vi "autonSample.vi"(0 "Auton Array":dbl[][](array[numeric]), 5 "LeftEncoder":dbl, 7 "RightEncoder":dbl, 11 "MeasuredHeading":dbl) -> (4 "Left Drive":dbl, 6 "Right Drive":dbl, 8 "Ramp ACT motor":dbl, 10 "Harvester":dbl, 13 "Shooter motor output":dbl, 14 "Turret Rotation":dbl, 15 "Convyeor":dbl)   [LabVIEW 2011]
uses:
  Robot Global Data.vi
panel:
  out "Primitive ID":i16
  out "Tzero":i64
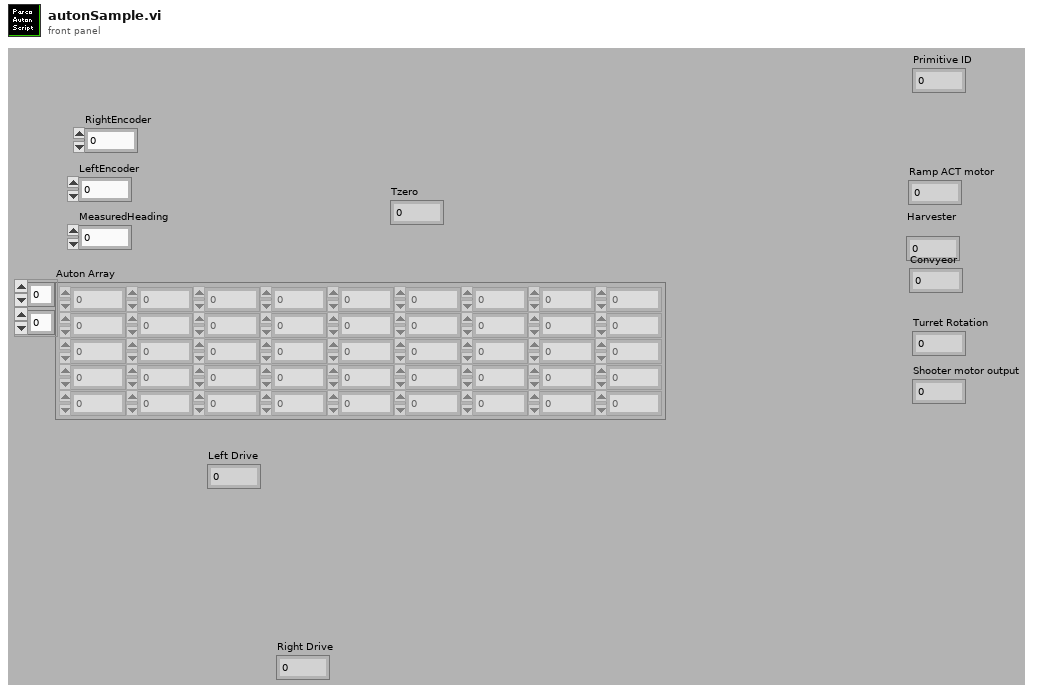
[diagram p1: front panel]
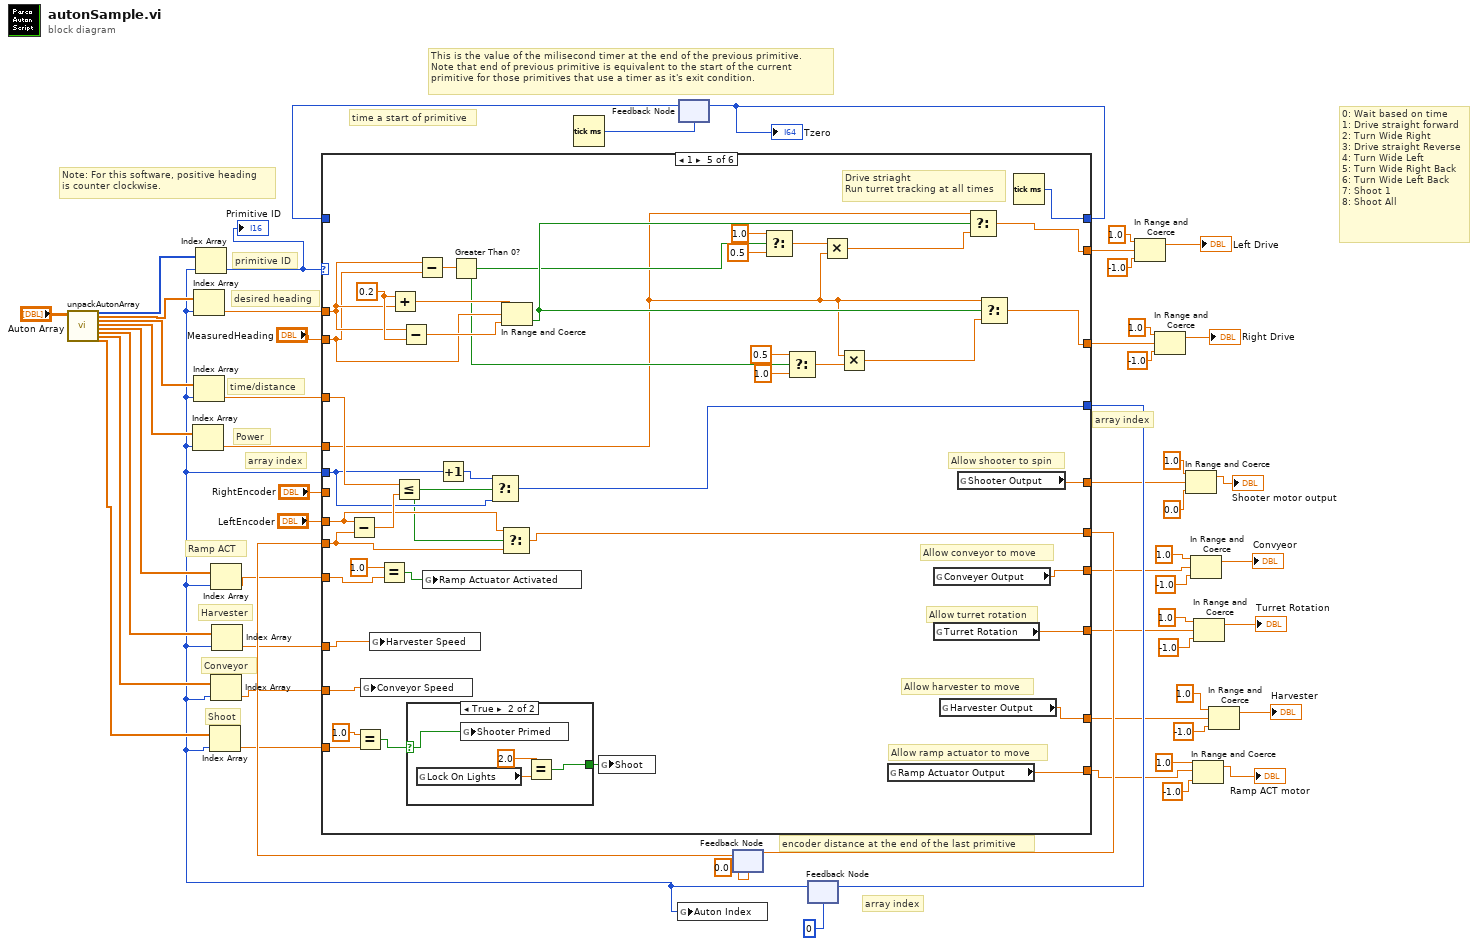
[diagram p0: block diagram]
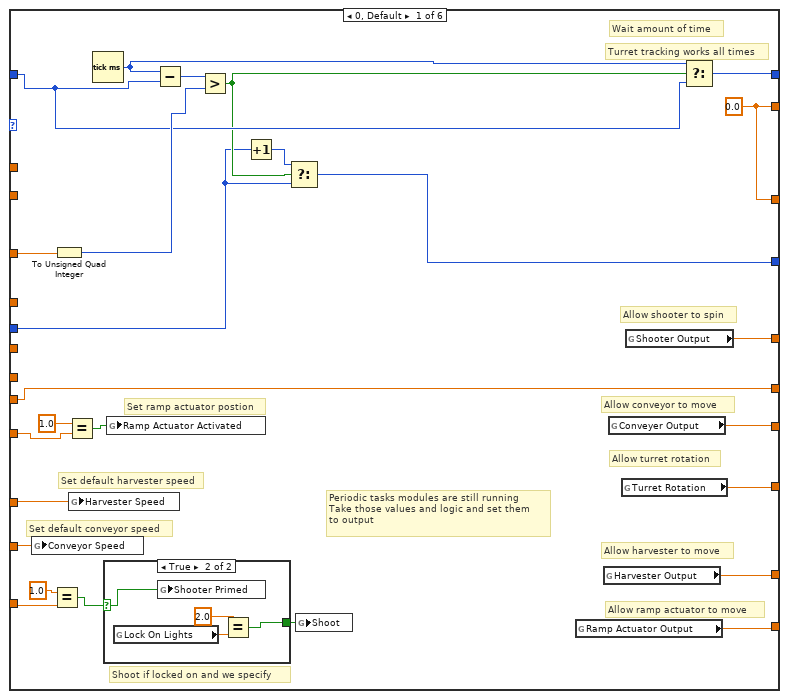
[diagram p2: hidden frame]
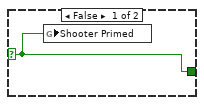
[diagram p3: hidden frame]
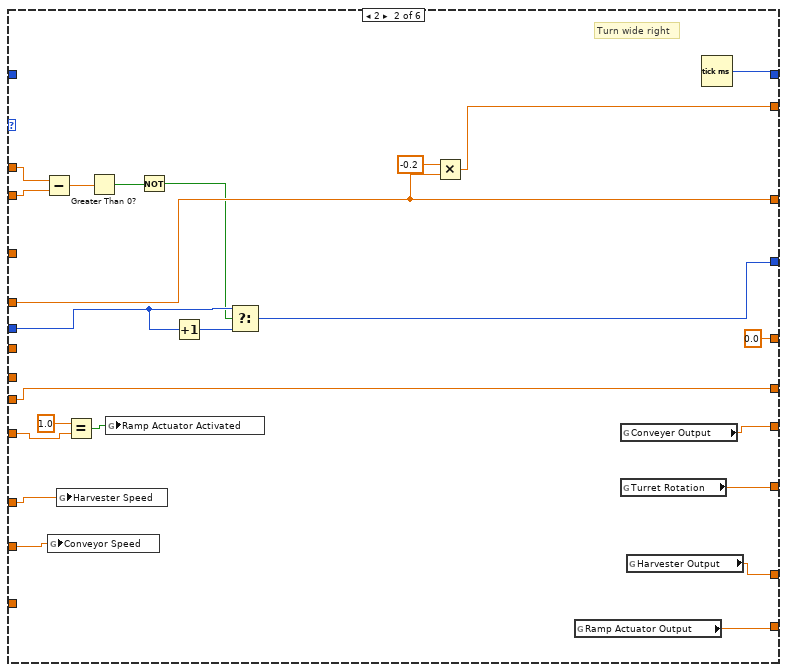
[diagram p4: hidden frame]
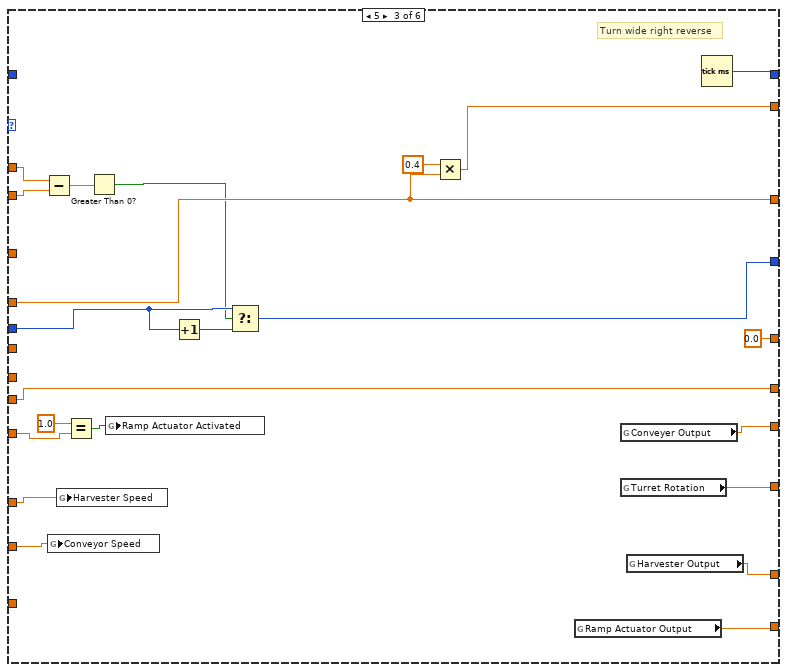
[diagram p5: hidden frame]
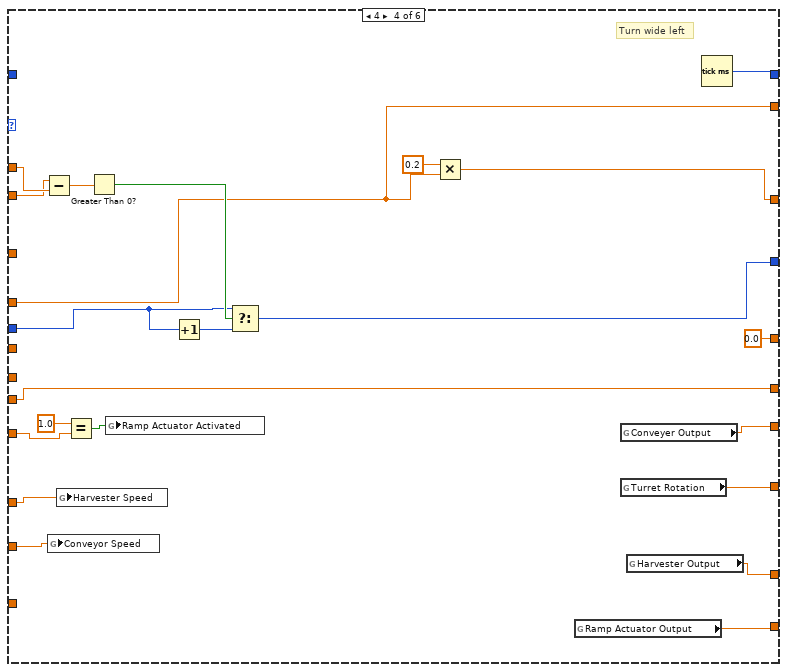
[diagram p6: hidden frame]
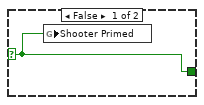
[diagram p7: hidden frame]
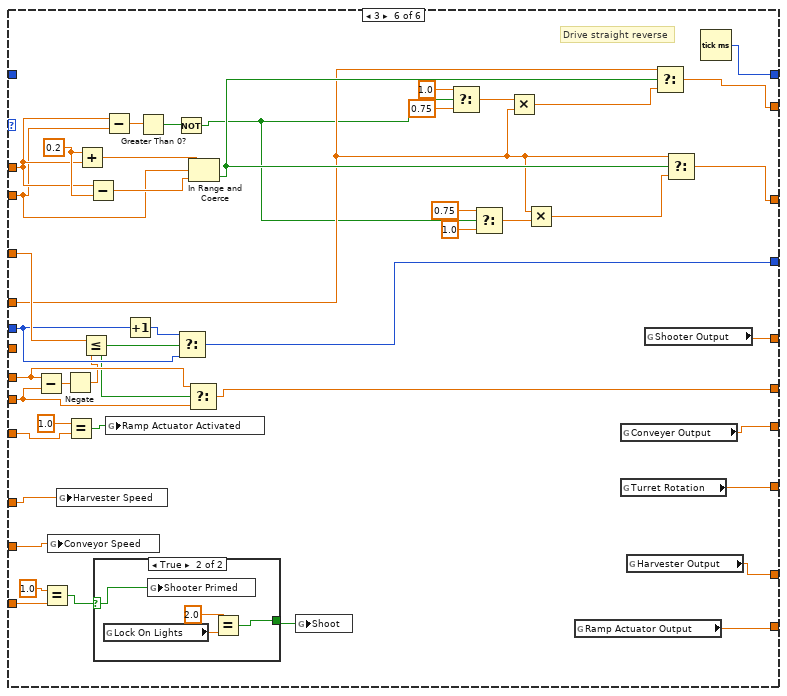
[diagram p8: hidden frame]
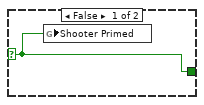
[diagram p9: hidden frame]
diagram:
  # "0: Wait based on time\n1: Drive straight forward\n2: Turn Wide Right\n3: Drive straight Reverse\n4: Turn Wide Left\n5: Turn Wide Right Back\n6: Turn Wide Left Back\n7: Shoot 1\n8: Shoot All"
  # "Shoot"
  # "Conveyor"
  # "Harvester"
  # "Ramp ACT"
  # "encoder distance at the end of the last primitive"
  # "Note: For this software, positive heading\nis counter clockwise."
  # "time a start of primitive"
  # "array index"
  # "array index"
  # "This is the value of the milisecond timer at the end of the previous primitive.\nNote that end of previous primitive is equivalent to the start of the current\nprimitive for those primitives that use a timer as it's exit condition."
  # "Power"
  # "array index"
  # "desired heading"
  # "primitive ID"
  # "time/distance"
  n1 = call "unpackAutonArray.vi"("all rows"="Auton Array") -> ("Primitive"=w56:i16[], "Desired Heading"=w16:dbl[], "Time/Distance"=w15:dbl[], "Power"=w14:dbl[], "Ramp Actuator"=w13:dbl[], "Harvester"=w12:dbl[], "Conveyor"=w11:dbl[], "Shoot"=w10:dbl[])  [unwired: 1 in, 18 out]
  n2 = Tick Count (ms)() -> (millisecond timer value=w51:u32)
  n3 = feedback #1(w51) -> (w55:u32)
  n4 = feedback #2(0.0 ("EncoderDistance")) -> (w39:dbl)
  n5 = feedback #3(0) -> (w8:i32)
  n6 = Index Array(array=w14, index=w8) -> (element=w53:dbl)
  n7 = Index Array(array=w16, index=w8) -> (element=w40:dbl)
  n8 = Index Array(array=w15, index=w8) -> (element=w54:dbl)
  n9 = Index Array(array=w56, index=w8) -> (element=w22:i16)
  "Primitive ID" <- w22
  n10 = Index Array(array=w10, index=w8) -> (element=w9:dbl)
  n11 = Index Array(array=w13, index=w8) -> (element=w21:dbl)
  n12 = Index Array(array=w11, index=w8) -> (element=w6:dbl)
  n13 = Index Array(array=w12, index=w8) -> (element=w7:dbl)
  n14 = case shown="1" w22 {
    tunnel: [w75 w91 w113 w139 w181 w232] -> w35
    tunnel: w8 -> [w76 w93 w115 w141 w183 w234]
    tunnel: [w83 w100 w122 w145 w159 w211] -> w41
    tunnel: w55 -> [w80 _ _ _ _ _]
    tunnel: w54 -> [w69 _ _ _ w184 w235]
    tunnel: w40 -> [_ w99 w121 w136 w172 w223]
    tunnel: [w74 w95 w117 w138 w158 w210] -> w49
    tunnel: [w74 w97 w119 w137 w157 w209] -> w42
    tunnel: w53 -> [_ w97 w119 w138 w161 w213]
    tunnel: "LeftEncoder" -> [_ _ _ _ w178 w229]
    tunnel: "MeasuredHeading" -> [_ w98 w120 w135 w171 w222]
    tunnel: [w68 w102 w124 w147 w180 w231] -> w36
    tunnel: w39 -> [w68 w102 w124 w147 w179 w230]
    tunnel: [w58 0.0 ("Shooter Output") 0.0 ("Shooter Output") 0.0 ("Shooter Output") w186 w236] -> w31
    tunnel: [w70 w108 w130 w152 w196 w245] -> w27
    tunnel: [w66 w104 w126 w149 w190 w240] -> w23
    tunnel: w21 -> [w63 w107 w129 w134 w193 w208]
    tunnel: [w71 w109 w131 w153 w197 w246] -> w20
    tunnel: w9 -> [w59 _ _ _ w194 w243]
    tunnel: w7 -> [w64 w106 w128 w151 w192 w242]
    tunnel: w6 -> [w65 w105 w127 w150 w191 w241]
    tunnel: [w67 w103 w125 w148 w189 w239] -> w2
    tunnel: "RightEncoder" -> [_ _ _ _ _ _]
    frame 0, Default {
      w74 = 0.0 ("Numeric")
      # "Periodic tasks modules are still running\nTake those values and logic and set them \nto output"
      # "Set ramp actuator postion"
      # "Set default harvester speed"
      # "Set default conveyor speed"
      # "Shoot if locked on and we specify"
      # "Allow ramp actuator to move"
      # "Allow harvester to move"
      # "Turret tracking works all times"
      # "Allow turret rotation"
      # "Allow conveyor to move"
      # "Allow shooter to spin"
      # "Wait amount of time"
      n15 = global write "Robot Global Data.vi" "Conveyor Speed"(w65) -> ()
      n16 = Equal?(x=1.0, y=w59) -> (x = y?=w61:bool)
      n17 = To Unsigned Quad Integer(1:w69) -> (0:w81:u64)
      n18 = Equal?(x=1.0, y=w63) -> (x = y?=w72:bool)
      n19 = global write "Robot Global Data.vi" "Harvester Speed"(w64) -> ()
      n20 = Tick Count (ms)() -> (millisecond timer value=w79:u32)
      n21 = case shown="True" w61 {
        selector: w61 -> [w84 w88]
        tunnel: [w84 w85] -> w60
        frame False {
          n22 = global write "Robot Global Data.vi" "Shooter Primed"(w84) -> ()
        }
        frame True {
          n23 = global read "Robot Global Data.vi" "Lock On Lights"() -> (w86:dbl)
          n24 = global write "Robot Global Data.vi" "Shooter Primed"(w88) -> ()
          n25 = Equal?(x=2.0, y=w86) -> (x = y?=w85:bool)
        }
      }
      n26 = global write "Robot Global Data.vi" "Ramp Actuator Activated"(w72) -> ()
      n27 = Subtract(x=w79, y=w80) -> (x-y=w82:u32)
      n28 = Greater?(x=w82, y=w81) -> (0:w78:bool)
      n29 = Increment(x=w76) -> (x+1=w77:i32)
      n30 = Select(t=w77, s=w78, f=w76) -> (s? t:f=w75:i32)
      n31 = global write "Robot Global Data.vi" "Shoot"(w60) -> ()
      n32 = global read "Robot Global Data.vi" "Ramp Actuator Output"() -> (w71:dbl)
      n33 = global read "Robot Global Data.vi" "Harvester Output"() -> (w66:dbl)
      n34 = global read "Robot Global Data.vi" "Conveyer Output"() -> (w67:dbl)
      n35 = global read "Robot Global Data.vi" "Turret Rotation"() -> (w70:dbl)
      n36 = global read "Robot Global Data.vi" "Shooter Output"() -> (w58:dbl)
      n37 = Select(t=w79, s=w78, f=w80) -> (s? t:f=w83:u32)
    }
    frame 2 {
      # "Turn wide right"
      n38 = Subtract(x=w99, y=w98) -> (x-y=w94:dbl)
      n39 = global write "Robot Global Data.vi" "Conveyor Speed"(w105) -> ()
      n40 = global write "Robot Global Data.vi" "Harvester Speed"(w106) -> ()
      n41 = Equal?(x=1.0, y=w107) -> (x = y?=w110:bool)
      n42 = Greater Than 0?(x=w94) -> (x > 0?=w90:bool)
      n43 = global write "Robot Global Data.vi" "Ramp Actuator Activated"(w110) -> ()
      n44 = Not(x=w90) -> (.not. x?=w89:bool)
      n45 = Increment(x=w93) -> (x+1=w92:i32)
      n46 = Select(t=w93, s=w89, f=w92) -> (s? t:f=w91:i32)
      n47 = Multiply(x=-0.2, y=w97) -> (x*y=w95:dbl)
      n48 = global read "Robot Global Data.vi" "Ramp Actuator Output"() -> (w109:dbl)
      n49 = global read "Robot Global Data.vi" "Conveyer Output"() -> (w103:dbl)
      n50 = global read "Robot Global Data.vi" "Turret Rotation"() -> (w108:dbl)
      n51 = global read "Robot Global Data.vi" "Harvester Output"() -> (w104:dbl)
      n52 = Tick Count (ms)() -> (millisecond timer value=w100:u32)
    }
    frame 5 {
      # "Turn wide right reverse"
      n53 = Subtract(x=w121, y=w120) -> (x-y=w116:dbl)
      n54 = global write "Robot Global Data.vi" "Conveyor Speed"(w127) -> ()
      n55 = global write "Robot Global Data.vi" "Harvester Speed"(w128) -> ()
      n56 = Equal?(x=1.0, y=w129) -> (x = y?=w132:bool)
      n57 = Greater Than 0?(x=w116) -> (x > 0?=w112:bool)
      n58 = global write "Robot Global Data.vi" "Ramp Actuator Activated"(w132) -> ()
      n59 = Increment(x=w115) -> (x+1=w114:i32)
      n60 = Select(t=w115, s=w112, f=w114) -> (s? t:f=w113:i32)
      n61 = Multiply(x=0.4, y=w119) -> (x*y=w117:dbl)
      n62 = global read "Robot Global Data.vi" "Ramp Actuator Output"() -> (w131:dbl)
      n63 = global read "Robot Global Data.vi" "Conveyer Output"() -> (w125:dbl)
      n64 = global read "Robot Global Data.vi" "Turret Rotation"() -> (w130:dbl)
      n65 = global read "Robot Global Data.vi" "Harvester Output"() -> (w126:dbl)
      n66 = Tick Count (ms)() -> (millisecond timer value=w122:u32)
    }
    frame 4 {
      # "Turn wide left"
      n67 = Subtract(x=w135, y=w136) -> (x-y=w143:dbl)
      n68 = global write "Robot Global Data.vi" "Conveyor Speed"(w150) -> ()
      n69 = global write "Robot Global Data.vi" "Harvester Speed"(w151) -> ()
      n70 = Equal?(x=1.0, y=w134) -> (x = y?=w154:bool)
      n71 = Greater Than 0?(x=w143) -> (x > 0?=w142:bool)
      n72 = global write "Robot Global Data.vi" "Ramp Actuator Activated"(w154) -> ()
      n73 = Increment(x=w141) -> (x+1=w140:i32)
      n74 = Select(t=w141, s=w142, f=w140) -> (s? t:f=w139:i32)
      n75 = Multiply(x=0.2, y=w138) -> (x*y=w137:dbl)
      n76 = global read "Robot Global Data.vi" "Ramp Actuator Output"() -> (w153:dbl)
      n77 = global read "Robot Global Data.vi" "Conveyer Output"() -> (w148:dbl)
      n78 = global read "Robot Global Data.vi" "Turret Rotation"() -> (w152:dbl)
      n79 = global read "Robot Global Data.vi" "Harvester Output"() -> (w149:dbl)
      n80 = Tick Count (ms)() -> (millisecond timer value=w145:u32)
    }
    frame 1 {
      w176 = 0.2 ("x")
      # "Allow ramp actuator to move"
      # "Allow harvester to move"
      # "Allow turret rotation"
      # "Allow conveyor to move"
      # "Allow shooter to spin"
      # "Drive striaght\nRun turret tracking at all times"
      n81 = Subtract(x=w178, y=w179) -> (x-y=w185:dbl)
      n82 = Equal?(x=1.0, y=w194) -> (x = y?=w188:bool)
      n83 = global write "Robot Global Data.vi" "Conveyor Speed"(w191) -> ()
      n84 = global write "Robot Global Data.vi" "Harvester Speed"(w192) -> ()
      n85 = Equal?(x=1.0, y=w193) -> (x = y?=w156:bool)
      n86 = Add(x=w176, y=w172) -> (x+y=w174:dbl)
      n87 = Less Or Equal?(x=w184, y=w185) -> (x <= y?=w177:bool)
      n88 = Subtract(x=w172, y=w176) -> (x-y=w175:dbl)
      n89 = case shown="True" w188 {
        selector: w188 -> [w199 w203]
        tunnel: [w199 w200] -> w187
        frame False {
          n90 = global write "Robot Global Data.vi" "Shooter Primed"(w199) -> ()
        }
        frame True {
          n91 = global read "Robot Global Data.vi" "Lock On Lights"() -> (w201:dbl)
          n92 = global write "Robot Global Data.vi" "Shooter Primed"(w203) -> ()
          n93 = Equal?(x=2.0, y=w201) -> (x = y?=w200:bool)
        }
      }
      n94 = Subtract(x=w172, y=w171) -> (x-y=w170:dbl)
      n95 = global write "Robot Global Data.vi" "Ramp Actuator Activated"(w156) -> ()
      n96 = Increment(x=w183) -> (x+1=w182:i32)
      n97 = Greater Than 0?(x=w170) -> (x > 0?=w169:bool)
      n98 = Select(t=w182, s=w177, f=w183) -> (s? t:f=w181:i32)
      n99 = Select(t=w178, s=w177, f=w179) -> (s? t:f=w180:dbl)
      n100 = In Range and Coerce(upper limit=w174, x=w171, lower limit=w175) -> (In Range?=w173:bool)  [unwired: 1 out]
      n101 = global write "Robot Global Data.vi" "Shoot"(w187) -> ()
      n102 = Select(t=1.0, s=w169, f=0.5) -> (s? t:f=w162:dbl)
      n103 = Select(t=0.5, s=w169, f=1.0) -> (s? t:f=w164:dbl)
      n104 = Multiply(x=w162, y=w161) -> (x*y=w160:dbl)
      n105 = Multiply(x=w161, y=w164) -> (x*y=w163:dbl)
      n106 = global read "Robot Global Data.vi" "Ramp Actuator Output"() -> (w197:dbl)
      n107 = global read "Robot Global Data.vi" "Conveyer Output"() -> (w189:dbl)
      n108 = global read "Robot Global Data.vi" "Turret Rotation"() -> (w196:dbl)
      n109 = global read "Robot Global Data.vi" "Harvester Output"() -> (w190:dbl)
      n110 = global read "Robot Global Data.vi" "Shooter Output"() -> (w186:dbl)
      n111 = Select(t=w161, s=w173, f=w160) -> (s? t:f=w158:dbl)
      n112 = Select(t=w161, s=w173, f=w163) -> (s? t:f=w157:dbl)
      n113 = Tick Count (ms)() -> (millisecond timer value=w159:u32)
    }
    frame 3 {
      w227 = 0.2 ("x")
      # "Drive straight reverse"
      n114 = Subtract(x=w229, y=w230) -> (x-y=w207:dbl)
      n115 = Equal?(x=1.0, y=w243) -> (x = y?=w238:bool)
      n116 = global write "Robot Global Data.vi" "Conveyor Speed"(w241) -> ()
      n117 = global write "Robot Global Data.vi" "Harvester Speed"(w242) -> ()
      n118 = Negate(x=w207) -> (-x=w206:dbl)
      n119 = Equal?(x=1.0, y=w208) -> (x = y?=w247:bool)
      n120 = Add(x=w227, y=w223) -> (x+y=w225:dbl)
      n121 = Less Or Equal?(x=w235, y=w206) -> (x <= y?=w228:bool)
      n122 = Subtract(x=w223, y=w227) -> (x-y=w226:dbl)
      n123 = case shown="True" w238 {
        selector: w238 -> [w249 w253]
        tunnel: [w249 w250] -> w237
        frame False {
          n124 = global write "Robot Global Data.vi" "Shooter Primed"(w249) -> ()
        }
        frame True {
          n125 = global read "Robot Global Data.vi" "Lock On Lights"() -> (w251:dbl)
          n126 = global write "Robot Global Data.vi" "Shooter Primed"(w253) -> ()
          n127 = Equal?(x=2.0, y=w251) -> (x = y?=w250:bool)
        }
      }
      n128 = Subtract(x=w223, y=w222) -> (x-y=w221:dbl)
      n129 = global write "Robot Global Data.vi" "Ramp Actuator Activated"(w247) -> ()
      n130 = Increment(x=w234) -> (x+1=w233:i32)
      n131 = Greater Than 0?(x=w221) -> (x > 0?=w205:bool)
      n132 = Not(x=w205) -> (.not. x?=w204:bool)
      n133 = Select(t=w233, s=w228, f=w234) -> (s? t:f=w232:i32)
      n134 = Select(t=w229, s=w228, f=w230) -> (s? t:f=w231:dbl)
      n135 = In Range and Coerce(upper limit=w225, x=w222, lower limit=w226) -> (In Range?=w224:bool)  [unwired: 1 out]
      n136 = global write "Robot Global Data.vi" "Shoot"(w237) -> ()
      n137 = Select(t=1.0, s=w204, f=0.75) -> (s? t:f=w214:dbl)
      n138 = Select(t=0.75, s=w204, f=1.0) -> (s? t:f=w216:dbl)
      n139 = Multiply(x=w214, y=w213) -> (x*y=w212:dbl)
      n140 = Multiply(x=w213, y=w216) -> (x*y=w215:dbl)
      n141 = global read "Robot Global Data.vi" "Ramp Actuator Output"() -> (w246:dbl)
      n142 = global read "Robot Global Data.vi" "Conveyer Output"() -> (w239:dbl)
      n143 = global read "Robot Global Data.vi" "Turret Rotation"() -> (w245:dbl)
      n144 = global read "Robot Global Data.vi" "Harvester Output"() -> (w240:dbl)
      n145 = global read "Robot Global Data.vi" "Shooter Output"() -> (w236:dbl)
      n146 = Select(t=w213, s=w224, f=w212) -> (s? t:f=w210:dbl)
      n147 = Select(t=w213, s=w224, f=w215) -> (s? t:f=w209:dbl)
      n148 = Tick Count (ms)() -> (millisecond timer value=w211:u32)
    }
  }
  "Tzero" <- w41
  n149 = global write "Robot Global Data.vi" "Auton Index"(w8) -> ()
  n150 = feedback-in #1(w41) -> ()
  n151 = feedback-in #2(w36) -> ()
  n152 = feedback-in #3(w35) -> ()
  n153 = In Range and Coerce(upper limit=1.0, x=w49, lower limit=-1.0) -> (coerced(x)=→"Left Drive":dbl)  [unwired: 1 out]
  n154 = In Range and Coerce(upper limit=1.0, x=w42, lower limit=-1.0) -> (coerced(x)=→"Right Drive":dbl)  [unwired: 1 out]
  n155 = In Range and Coerce(upper limit=1.0, x=w31, lower limit=0.0) -> (coerced(x)=→"Shooter motor output":dbl)  [unwired: 1 out]
  n156 = In Range and Coerce(upper limit=1.0, x=w2, lower limit=-1.0) -> (coerced(x)=→"Convyeor":dbl)  [unwired: 1 out]
  n157 = In Range and Coerce(upper limit=1.0, x=w20, lower limit=-1.0) -> (coerced(x)=→"Ramp ACT motor":dbl)  [unwired: 1 out]
  n158 = In Range and Coerce(upper limit=1.0, x=w27, lower limit=-1.0) -> (coerced(x)=→"Turret Rotation":dbl)  [unwired: 1 out]
  n159 = In Range and Coerce(upper limit=1.0, x=w23, lower limit=-1.0) -> (coerced(x)=→"Harvester":dbl)  [unwired: 1 out]
